vi "Create Events.vi"(7 "error in":errorcluster, 10 "Message Pump in":refnum<class "Message Pump.lvclass">) -> (0 "error out":errorcluster, 2 "Event Registration Refnum":refnum<event-registration>, 3 "Message Pump out":refnum<class "Message Pump.lvclass">)   [LabVIEW 2023, in "GUI.lvlib" / "Message Pump.lvclass"]
doc: "Creates the events required for the Worker's QMH's EHL."
uses:
  Message Pump.lvclass
  Message Pump.lvclass/Message Pump.ctl
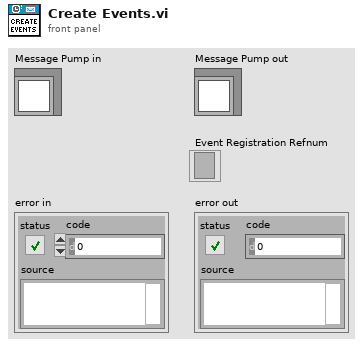
[diagram p1: front panel]
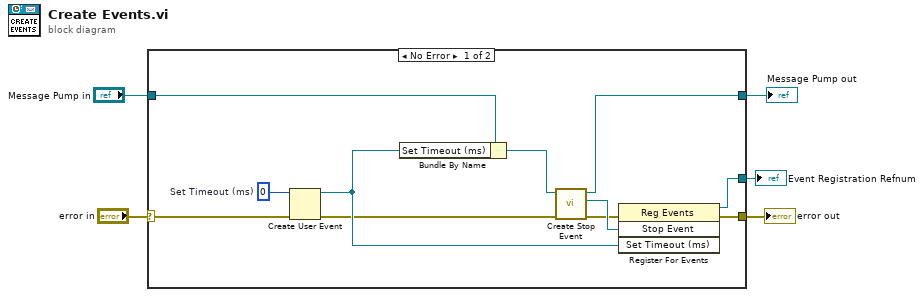
[diagram p0: block diagram]
diagram:
  n1 = case shown="No Error" "error in" {
    selector: "error in" -> [w7 w18]
    tunnel: [w16 w18] -> w5
    tunnel: [w13 _] -> w1
    tunnel: "Message Pump in" -> [w9 w17]
    tunnel: [w10 w17] -> w2
    frame No Error {
      w14 = 0  # Set Timeout (ms)
      n2 = Create User Event(user event datatype=w14, error in=w7) -> (user event=w15:refnum<user-event>, error out=w6:errorcluster)
      n3 = Bundle By Name(cluster=w9, "Set Timeout (ms)"=w15) -> (w8:refnum<class "Message Pump.lvclass">)
      n4 = call-dynamic "Create Stop Event.vi"("error in"=w6, "Worker"=w8) -> ("error out"=w11:errorcluster, "Stop Event"=w12:refnum<user-event>, "Worker out"=w10:refnum<class "Message Pump.lvclass">)  [unwired: 7 in]
      n5 = register-events(error in=w11, w12, w15) -> (reference out=w13:refnum<event-registration>, error out=w16:errorcluster)  [unwired: 1 in]
    }
    frame Error {
    }
  }
  "error out" <- w5
  "Message Pump out" <- w2
  "Event Registration Refnum" <- w1
